vi "CC Alarm Object.vi"(8 "error in (no error)":errorcluster, 9 "Alarm":T1, 10 "Source":string, 11 "Alarm Action":T2) -> (0 "error out":errorcluster, 2 "Alarm List":T1[](array[typedef]), 3 "Alarm?":bool)   [LabVIEW 2021]
uses:
  typedefs/CC cluster Alarm Data.ctl
  typedefs/CC enum Alarm Action.ctl
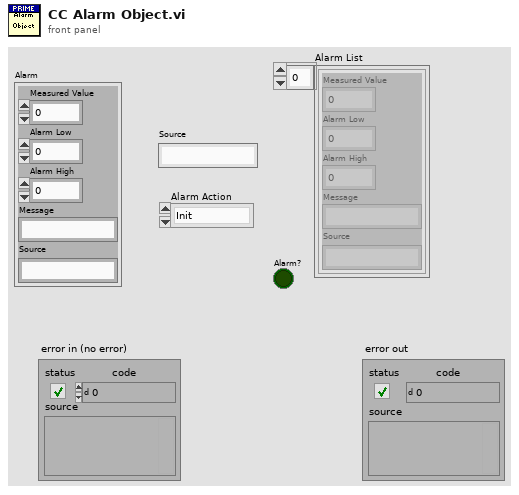
[diagram p1: front panel]
types:
  T1 = typedef "CC cluster Alarm Data.ctl" = cluster{"Measured Value":dbl, "Alarm Low":dbl, "Alarm High":dbl, "Message":string, "Source":string}
  T2 = typedef "CC enum Alarm Action.ctl" = enum16{"Init", "Add Alarm", "Get Alarms", "Clear Alarm", "Clear All Alarms"}
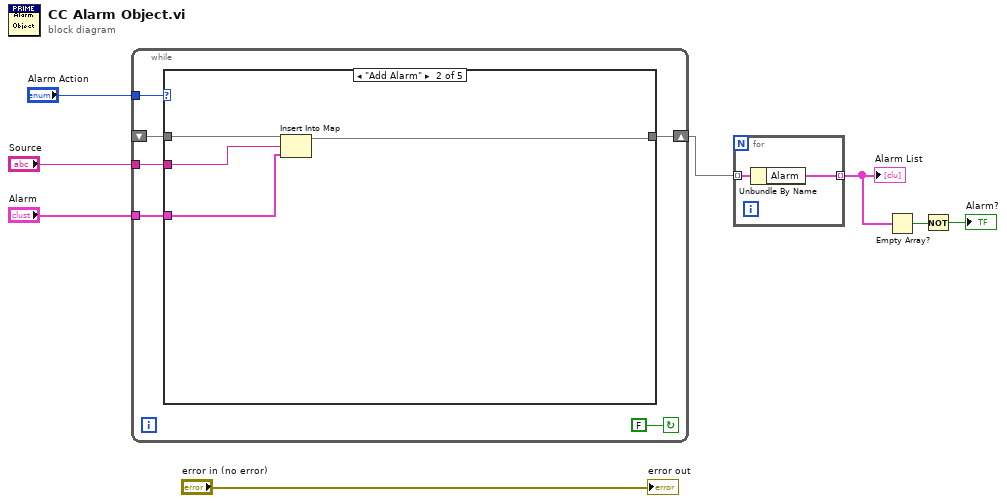
[diagram p0: block diagram]
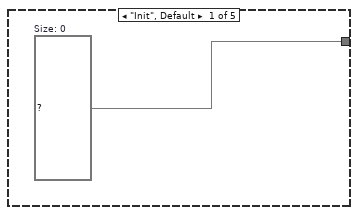
[diagram p2: hidden frame]
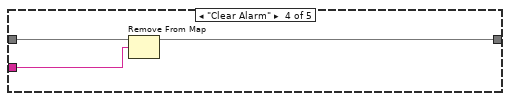
[diagram p4: hidden frame]
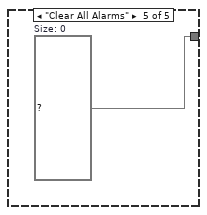
[diagram p5: hidden frame]
diagram:
  n1 = while {
    tunnel: "Alarm Action" -> [w13]
    shift-right: [w12] -> w4
    shift-left: _ -> [w11]
    tunnel: "Source" -> [w10]
    tunnel: "Alarm" -> [w9]
    stop <- FALSE continue-if-true
    n2 = case shown="\"Add Alarm\"" w13 {
      tunnel: [w15 w16 w20 w21 w24] -> w12
      tunnel: w11 -> [_ w19 w20 w23 _]
      tunnel: w10 -> [_ w18 _ w22 _]
      tunnel: w9 -> [_ w17 _ _ _]
      frame "Init", Default {
        w15 = map{string, T1} {}  # Size: 0
      }
      frame "Add Alarm" {
        n3 = Insert Into Map(map in=w19, key=w18, value=w17) -> (map out=w16:map{string, T1})  [unwired: 2 out]
      }
      frame "Get Alarms" {
      }
      frame "Clear Alarm" {
        n4 = Remove From Map(10:w22, 11:w23) -> (3:w21:map{string, T1})  [unwired: 2 out]
      }
      frame "Clear All Alarms" {
        w24 = map{string, T1} {}  # Size: 0
      }
    }
  }
  n5 = for {
    tunnel: w4 -> [w26] mode=indexing
    tunnel: [w25] -> w3 mode=indexing
    n6 = Unbundle By Name(w26) -> ("Alarm"=w25:T1)
  }
  "Alarm List" <- w3
  n7 = Empty Array?(array=w3) -> (empty?=w2:bool)
  n8 = Not(x=w2) -> (.not. x?=→"Alarm?":bool)
  "error out" <- "error in (no error)"
